vi "CMN_GetBuffers.vi"(10 "deftransferbufsize":u32=131072, 11 "database name":string="DBS") -> (2 "BuffersDimensions":T1={"TotalPixels"=0, "Total image bytes"=0, "Total Phys Buffers"=0, "virtual buf pixels"=0, "virtual bytes size"=0, "Remaining piece"=0, "Transfer_Buf_size"=131072})   [LabVIEW 2016]
uses:
  CMN_Buffers.ctl
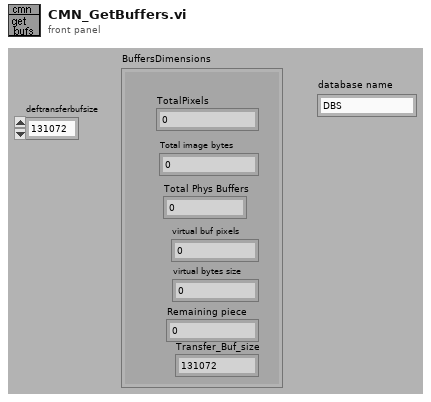
[diagram p1: front panel]
types:
  T1 = typedef "CMN_Buffers.ctl" = cluster{"TotalPixels":u32, "Total image bytes":u32, "Total Phys Buffers":u32, "virtual buf pixels":u32, "virtual bytes size":u32, "Remaining piece":u32, "Transfer_Buf_size":u32}
  T2 = typedef "DatabaseHand_RefNum.ctl" = refnum<vi>
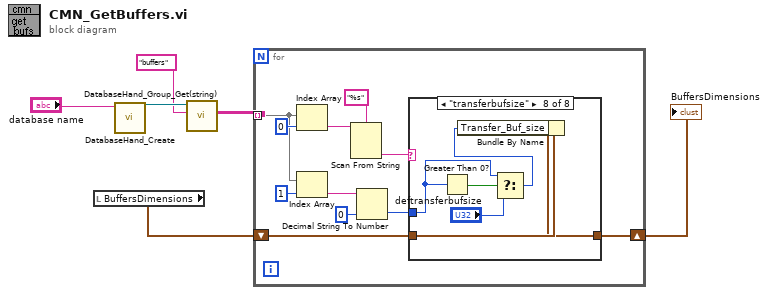
[diagram p0: block diagram]
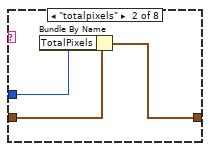
[diagram p3: hidden frame]
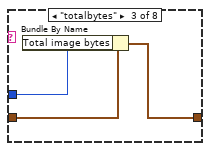
[diagram p4: hidden frame]
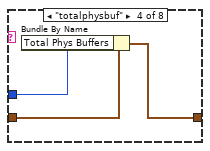
[diagram p5: hidden frame]
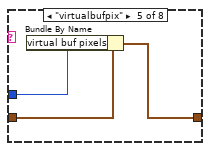
[diagram p6: hidden frame]
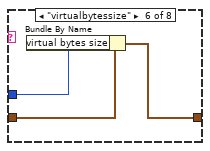
[diagram p7: hidden frame]
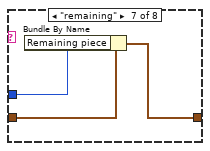
[diagram p8: hidden frame]
diagram:
  n1 = local read "BuffersDimensions"() -> (w1:T1)
  n2 = call "DatabaseHand_Create.vi"("Name"="database name") -> ("Database RefNum out"=w5:T2)  [unwired: 1 in, 9 out]
  n3 = call "DatabaseHand_Group_Get(string).vi"("group"="buffers", "Database RefNum in"=w5) -> ("group array"=w3:string[][])  [unwired: 1 in, 8 out]
  n4 = for {
    tunnel: w3 -> [w15] mode=indexing
    shift-right: [w8] -> w2
    shift-left: w1 -> [w11]
    n5 = Index Array(array=w15, index=0) -> (element=w14:string)
    n6 = Index Array(array=w15, index=1) -> (element=w10:string)
    n7 = Scan From String(format string="%s", input string=w14) -> (output 1=w12:string)  [unwired: 2 in, 4 out]
    n8 = Decimal String To Number(string=w10, default (0L)=u32 0) -> (number=w9:u32)  [unwired: 2 out]
    n9 = case shown="\"transferbufsize\"" w12 {
      tunnel: w11 -> [w18 w21 w24 w27 w30 w33 w36 w42]
      tunnel: w9 -> [_ w20 w23 w26 w29 w32 w35 w38]
      tunnel: [w18 w19 w22 w25 w28 w31 w34 w41] -> w8
      frame Default {
      }
      frame "totalpixels" {
        n10 = Bundle By Name(cluster=w21, "TotalPixels"=w20) -> (w19:T1)
      }
      frame "totalbytes" {
        n11 = Bundle By Name(cluster=w24, "Total image bytes"=w23) -> (w22:T1)
      }
      frame "totalphysbuf" {
        n12 = Bundle By Name(cluster=w27, "Total Phys Buffers"=w26) -> (w25:T1)
      }
      frame "virtualbufpix" {
        n13 = Bundle By Name(cluster=w30, "virtual buf pixels"=w29) -> (w28:T1)
      }
      frame "virtualbytessize" {
        n14 = Bundle By Name(cluster=w33, "virtual bytes size"=w32) -> (w31:T1)
      }
      frame "remaining" {
        n15 = Bundle By Name(cluster=w36, "Remaining piece"=w35) -> (w34:T1)
      }
      frame "transferbufsize" {
        n16 = Greater Than 0?(x=w38) -> (x > 0?=w39:bool)
        n17 = Select(t=w38, s=w39, f="deftransferbufsize") -> (s? t:f=w37:u32)
        n18 = Bundle By Name(cluster=w42, "Transfer_Buf_size"=w37) -> (w41:T1)
      }
    }
  }
  "BuffersDimensions" <- w2
